vi "Set Serial Port.vi"(8 "error in (no error)":errorcluster, 10 "Serial Port":string, 11 "Serial Device in":refnum<class "Serial Device.lvclass">) -> (0 "error out":errorcluster, 3 "Serial Device out":refnum<class "Serial Device.lvclass">)   [LabVIEW 2017, in "Serial Device.lvclass"]
uses:
  Serial Device.lvclass
  Serial Device.lvclass/Serial Device.ctl
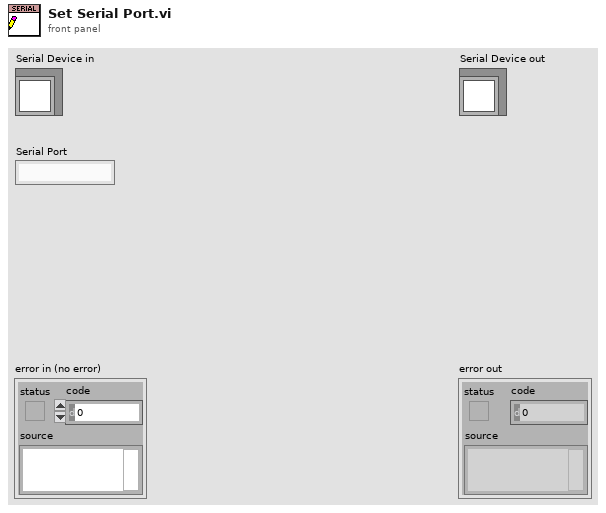
[diagram p1: front panel]
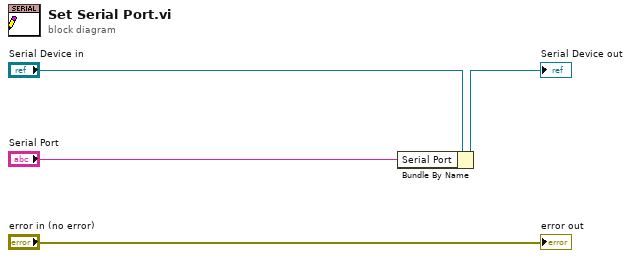
[diagram p0: block diagram]
diagram:
  n1 = Bundle By Name(cluster="Serial Device in", "Serial Port"="Serial Port") -> (→"Serial Device out":refnum<class "Serial Device.lvclass">)
  "error out" <- "error in (no error)"
